vi "Periodic Tasks.vi"(8 "error in":errorcluster) -> ()   [LabVIEW 2013]
doc: "This VI runs in parallel to other tasks. It can contain as many user-defined periodic loops as you need. These can carry out PID or other sorts of timed response."
uses:
  RefnameEnum.ctl
  ActionEnum.ctl
  <vilib>/Rock Robotics/SystemInterfaces/Utilities/FPGA_UtilitiesLED Source.ctl
  <vilib>/Rock Robotics/SystemInterfaces/Utilities/FPGA_UtilitiesLED State.ctl
  TankDriveInstruction.ctl
  Robot Global Data.vi
  <vilib>/Rock Robotics/WPI/Compressor/WPI_CompressorGetSetRefNum.vi
  <vilib>/Rock Robotics/WPI/RobotDrive/WPI_RobotDriveGetSetRefNum.vi
panel:
  out "MainQueue size":i32
  out "TankDriveQueue size":i32
  out "IDNum Diff":i32
  out "MainQueue\nInterval":u32
  out "TankDrive\nInterval":u32
  out "ProcessInput\nInterval":u32
  out "TeleopInterval":i32
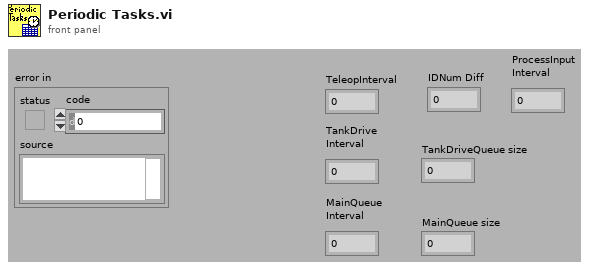
[diagram p1: front panel]
types:
  T1 = typedef "ActionEnum.ctl" = enum16{"Init", "SetValue"}
  T2 = typedef "RefnameEnum.ctl" = enum16{"FireLauncher", "Climber", "Shield", "TankDrive", "DriveEncoderL", "DriveEncoderR", "LauncherMotorRPM", "LauncherEncoderAnalog", "LauncherEncoderRPM", "ShooterLS", "DriveAlignLSLeft", "DriveAlignLSRight", "ClimbingLS", "LauncherEncoderAngle", "LauncherMotorAngle", "Gamepad1", "Gamepad2", "Compressor", "ClimbWeightSol3", "ClimbWeightSol4"}
  T3 = typedef "WPI_SolenoidDevRef.ctl" = cluster{"DevStatus":errorcluster, "Solenoid Module":T4, "Forward Solenoid Channel":T5, "Reverse Solenoid Channel":T5}
  T4 = typedef "FPGA_TypedefSolenoidModule.ctl" = enum16{"Solenoid Module 1", "Solenoid Module 2"}
  T5 = typedef "WPI_SolenoidChannel.ctl" = enum8{"Solenoid 1", "Solenoid 2", "Solenoid 3", "Solenoid 4", "Solenoid 5", "Solenoid 6", "Solenoid 7", "Solenoid 8", "Invalid"}
  T6 = typedef "WPI_RobotDriveDevRef.ctl" = cluster{"DevStatus":errorcluster, "Motors[]":T7[], "Square Inputs":bool, "Max Output":dbl, "Isochronous":bool}
  T7 = typedef "WPI_MotorControlDeviceRef.ctl" = cluster{"DeviceStatus":errorcluster, "Type":enum16{"PWM", "CAN"}, "PWM":cluster{"Digital Module":T8, "PWM Channel":T9, "DeadBand":T10}, "CAN":cluster{"Device Number":u8, "Control Mode":T11, "Semaphore":T12, "Max Vout":dbl}, "Invert":bool, "TransformRef":T13, "InvTransformRef":T13}
  T8 = typedef "FPGA_TypedefDigitalModule.ctl" = enum16{"Digital Module 1", "Digital Module 2"}
  T9 = typedef "FPGA_DIOPWMChannel.ctl" = enum8{"PWM 1", "PWM 2", "PWM 3", "PWM 4", "PWM 5", "PWM 6", "PWM 7", "PWM 8", "PWM 9", "PWM 10", "Invalid"}
  T10 = typedef "WPI_PWMDeadband.ctl" = cluster{"Name":string, "maxPositivePwm":i32, "minPositivePwm":i32, "centerPwm":i32, "maxNegativePwm":i32, "minNegativePwm":i32, "angularRange":u16}
  T11 = typedef "WPI_CANJaguar_ControlMode.ctl" = enum8{"Percent VBus", "Current", "Speed", "Position", "Voltage"}
  T12 = typedef "Semaphore RefNum" = refnum<k1>
  T13 = typedef "WPI_PWMTransform_ConPane.ctl" = refnum<vi>
  T14 = typedef "WPI_CompressorDevRef.ctl" = cluster{"DevStatus":errorcluster, "DigitalInputDevRef":T15, "RelayDevRef":T17}
  T15 = typedef "WPI_DigitalInputDevRef.ctl" = cluster{"DevStatus":errorcluster, "DIO Channel":T16, "Digital Module":T8}
  T16 = typedef "FPGA_DIOChannel.ctl" = enum8{"DIO 1", "DIO 2", "DIO 3", "DIO 4", "DIO 5", "DIO 6", "DIO 7", "DIO 8", "DIO 9", "DIO 10", "DIO 11", "DIO 12", "DIO 13", "DIO 14", "Invalid"}
  T17 = typedef "WPI_RelayDevRef.ctl" = cluster{"DevStatus":errorcluster, "Relay Channel":T18, "Digital Module":T8, "Relay Direction":T19}
  T18 = typedef "FPGA_DIORelayChannel.ctl" = enum8{"Relay 1", "Relay 2", "Relay 3", "Relay 4", "Relay 5", "Relay 6", "Relay 7", "Relay 8", "Invalid"}
  T19 = typedef "WPI_RelayDirection.ctl" = enum16{"Both directions", "Forward only", "Reverse only"}
  T20 = typedef "QueueInstruction.ctl" = cluster{"Data":variant, "Subsystem":T21, "Action":T1}
  T21 = typedef "SubsystemEnum.ctl" = enum16{"TankDrive", "FirePneumatic", "Climber", "ClimbWeight", "ShooterAngle"}
  T22 = typedef "TankDriveInstruction.ctl" = cluster{"LeftMotorValue":dbl, "RightMotorValue":dbl, "HalfSpeed":bool}
  T23 = typedef "FPGA_UtilitiesLED State.ctl" = enum16{"Off", "On", "Toggle"}
  T24 = typedef "FPGA_UtilitiesLED Source.ctl" = enum16{"User LED", "FPGA LED"}
  T25 = typedef "TeleopData.ctl" = cluster{"cTankDriveLeft":dbl, "cTankDriveRight":dbl, "cHalfSpeed":bool, "cClimbWeight":bool, "cClimbStart":bool, "cRpmControl":dbl, "cAngleControl":dbl, "cQuickShoot":bool, "cLauncherWheel":bool, "cFirePneumatic":bool, "cPresetLow":bool, "cPresetHigh":bool, "cPresetClimbLow":bool, "cPresetClimbHigh":bool, "cLauncherAngle":bool, "cResetAngleEncoder":bool, "IDNum":i32, "TeleopInterval":i32}
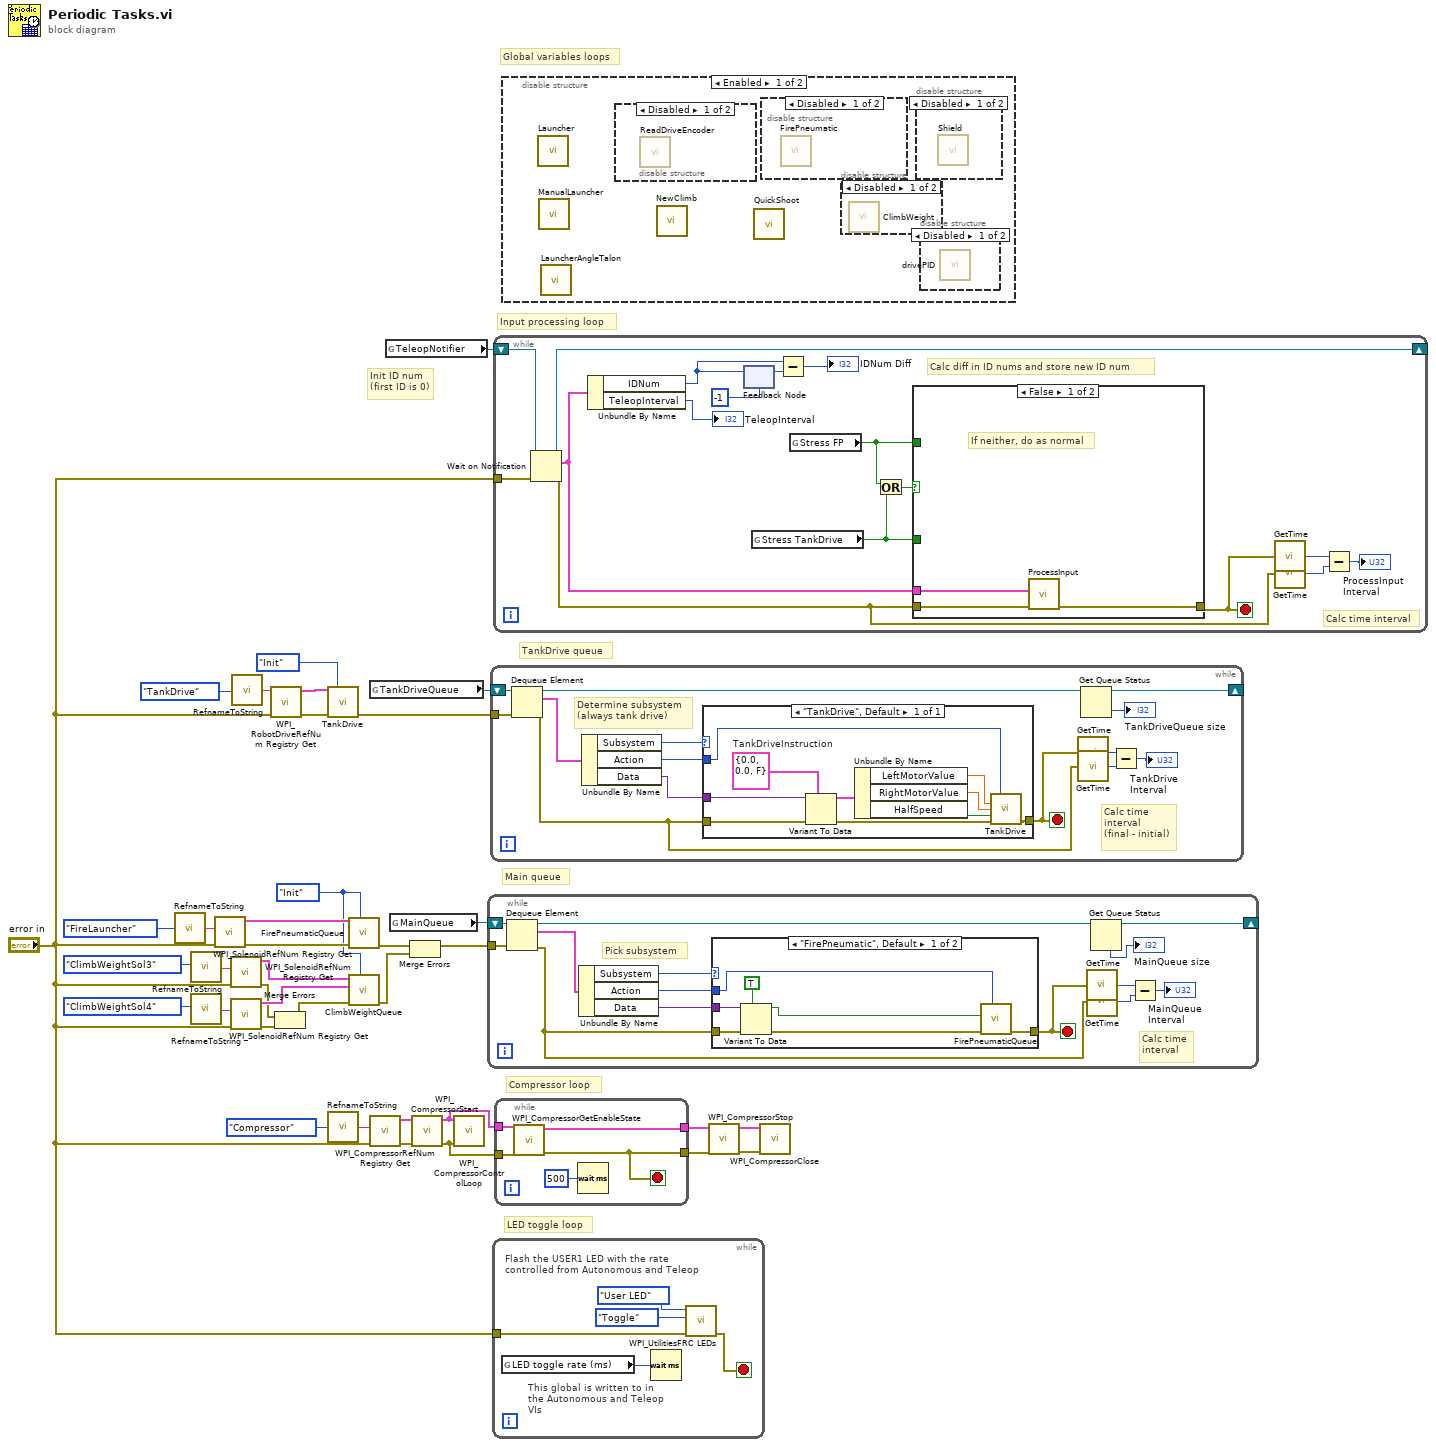
[diagram p0: block diagram]
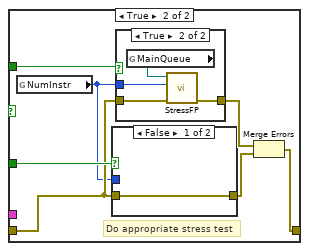
[diagram p2: hidden frame]
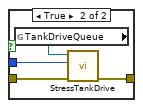
[diagram p3: hidden frame]
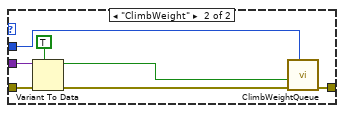
[diagram p5: hidden frame]
diagram:
  w2 = ActionEnum."Init" ("Action")
  # "Init ID num\n(first ID is 0)"
  # "Global variables loops"
  # "LED toggle loop"
  # "Compressor loop"
  # "Main queue"
  # "Input processing loop"
  # "TankDrive queue"
  n1 = call "RefnameToString.vi"("Enum"=RefnameEnum."FireLauncher") -> ("Refname"=w25:string)
  n2 = call "RefnameToString.vi"("Enum"=RefnameEnum."ClimbWeightSol3") -> ("Refname"=w11:string)
  n3 = call "RefnameToString.vi"("Enum"=RefnameEnum."ClimbWeightSol4") -> ("Refname"=w9:string)
  n4 = call <vilib>:"WPI_SolenoidRefNum Registry Get.vi"("error in (no error)"="error in", "refnum name"=w25) -> ("error out"=w18:errorcluster, "SolenoidDevRef"=w19:T3)  [unwired: 8 in]
  n5 = call <vilib>:"WPI_SolenoidRefNum Registry Get.vi"("error in (no error)"="error in", "refnum name"=w11) -> ("error out"=w4:errorcluster, "SolenoidDevRef"=w7:T3)  [unwired: 8 in]
  n6 = call <vilib>:"WPI_SolenoidRefNum Registry Get.vi"("error in (no error)"="error in", "refnum name"=w9) -> ("error out"=w5:errorcluster, "SolenoidDevRef"=w6:T3)  [unwired: 8 in]
  n7 = call "RefnameToString.vi"("Enum"=RefnameEnum."TankDrive") -> ("Refname"=w30:string)
  n8 = call <vilib>:"WPI_RobotDriveRefNum Registry Get.vi"("error in (no error)"="error in", "refnum name"=w30) -> ("error out"=w21:errorcluster, "RobotDriveDevRef"=w22:T6)  [unwired: 8 in]
  n9 = Merge Errors(w4, w5) -> (w3:errorcluster)
  n10 = call "TankDrive.vi"("RobotDriveDevRef"=w22, "Action"=ActionEnum."Init", "Error In (no error)"=w21) -> ("Error Out"=w20:errorcluster)  [unwired: 12 in]
  n11 = call "RefnameToString.vi"("Enum"=RefnameEnum."Compressor") -> ("Refname"=w32:string)
  n12 = call "FirePneumaticQueue.vi"("Action"=w2, "error in (no error)"=w18, "SolenoidDevRef"=w19) -> ("error out"=w15:errorcluster)  [unwired: 8 in]
  n13 = call "ClimbWeightQueue.vi"("Action"=w2, "error in (no error)"=w3, "ClimbWeightSol4"=w6, "ClimbWeightSol3"=w7) -> ("error out"=w13:errorcluster)  [unwired: 7 in]
  n14 = global read "Robot Global Data.vi" "TankDriveQueue"() -> (w28:refnum<queue>)
  n15 = call <vilib>:"WPI_CompressorRefNum Registry Get.vi"("error in (no error)"="error in", "refnum name"=w32) -> ("error out"=w24:errorcluster, "CompressorDevRef"=w37:T14)  [unwired: 8 in]
  n16 = global read "Robot Global Data.vi" "TeleopNotifier"() -> (w29:refnum<notifier>)
  n17 = global read "Robot Global Data.vi" "MainQueue"() -> (w27:refnum<queue>)
  n18 = Merge Errors(w15, w13) -> (w14:errorcluster)
  n19 = call <vilib>:"WPI_CompressorStart.vi"("error in (no error)"=w24, "CompressorDevRef"=w37) -> ("error out"=w23:errorcluster, "CompressorDevRef"=w36:T14)  [unwired: 8 in]
  n20 = call <vilib>:"WPI_CompressorControlLoop.vi"("error in (no error)"=w23, "CompressorDevRef"=w36) -> ()  [unwired: 10 in]
  n21 = while {
    shift-right: [w41] -> _
    shift-left: w27 -> [w51]
    tunnel: w14 -> [w49]
    stop <- w44 stop-if-true
    # "Calc time\ninterval"
    # "Pick subsystem"
    n22 = Dequeue Element(queue=w51, error in (no error)=w49) -> (queue out=w42:refnum<queue>, element=w50:T20, error out=w43:errorcluster)  [unwired: 1 in, 1 out]
    n23 = Unbundle By Name(w50) -> ("Subsystem"=w48:T21, "Action"=w38:T1, "Data"=w39:variant)
    n24 = case shown="\"FirePneumatic\", Default" w48 {
      tunnel: w43 -> [w54 w64]
      tunnel: [w57 w65] -> w44
      tunnel: w39 -> [w55 w62]
      tunnel: w38 -> [w52 w59]
      frame "FirePneumatic", Default {
        n25 = Variant To Data(error in=w54, type=TRUE, Variant=w55) -> (data=w56:bool, error out=w53:errorcluster)
        n26 = call "FirePneumaticQueue.vi"("Action"=w52, "error in (no error)"=w53, "On/off?"=w56) -> ("error out"=w57:errorcluster)  [unwired: 8 in]
      }
      frame "ClimbWeight" {
        n27 = Variant To Data(error in=w64, type=TRUE, Variant=w62) -> (data=w60:bool, error out=w63:errorcluster)
        n28 = call "ClimbWeightQueue.vi"("Action"=w59, "error in (no error)"=w63, "Swing Out?"=w60) -> ("error out"=w65:errorcluster)  [unwired: 8 in]
      }
    }
    n29 = call "GetTime.vi"("error in"=w44) -> ("Time"=w46:u32)
    n30 = call "GetTime.vi"("error in"=w43) -> ("Time"=w47:u32)
    n31 = Get Queue Status(queue=w42) -> (queue out=w41:refnum<queue>, # elements in queue=→"MainQueue size":i32)  [unwired: 2 in, 6 out]
    n32 = Subtract(x=w46, y=w47) -> (x-y=→"MainQueue\nInterval":u32)
  }
  n33 = while {
    shift-right: [w69] -> _
    shift-left: w28 -> [w79]
    tunnel: w20 -> [w76]
    stop <- w74 stop-if-true
    # "Calc time\ninterval\n(final - initial)"
    # "Determine subsystem\n(always tank drive)"
    n34 = Dequeue Element(queue=w79, error in (no error)=w76) -> (queue out=w70:refnum<queue>, element=w78:T20, error out=w75:errorcluster)  [unwired: 1 in, 1 out]
    n35 = Unbundle By Name(w78) -> ("Subsystem"=w77:T21, "Action"=w66:T1, "Data"=w67:variant)
    n36 = case shown="\"TankDrive\", Default" w77 {
      tunnel: w75 -> [w86]
      tunnel: [w85] -> w74
      tunnel: w67 -> [w81]
      tunnel: w66 -> [w80]
      frame "TankDrive", Default {
        w89 = T22 {"LeftMotorValue"=0.0, "RightMotorValue"=0.0, "HalfSpeed"=FALSE}  # TankDriveInstruction
        n37 = Variant To Data(error in=w86, type=w89, Variant=w81) -> (data=w88:T22, error out=w87:errorcluster)
        n38 = Unbundle By Name(w88) -> ("LeftMotorValue"=w82:dbl, "RightMotorValue"=w83:dbl, "HalfSpeed"=w84:bool)
        n39 = call "TankDrive.vi"("Action"=w80, "Left Motor Value"=w82, "Right Motor Value"=w83, "HalfSpeed"=w84, "Error In (no error)"=w87) -> ("Error Out"=w85:errorcluster)  [unwired: 10 in]
      }
    }
    n40 = call "GetTime.vi"("error in"=w74) -> ("Time"=w72:u32)
    n41 = call "GetTime.vi"("error in"=w75) -> ("Time"=w71:u32)
    n42 = Get Queue Status(queue=w70) -> (queue out=w69:refnum<queue>, # elements in queue=→"TankDriveQueue size":i32)  [unwired: 2 in, 6 out]
    n43 = Subtract(x=w72, y=w71) -> (x-y=→"TankDrive\nInterval":u32)
  }
  n44 = while {
    tunnel: "error in" -> [w91]
    stop <- w90 stop-if-true
    # "This global is written to in the Autonomous and Teleop VIs"
    # "Flash the USER1 LED with the rate controlled from Autonomous and Teleop"
    n45 = global read "Robot Global Data.vi" "LED toggle rate (ms)"() -> (w92:u32)
    n46 = Wait (ms)(milliseconds to wait=w92) -> ()  [unwired: 1 out]
    n47 = call <vilib>:"WPI_UtilitiesFRC LEDs.vi"("error in (no error)"=w91, "State"=FPGA_UtilitiesLED_State."Toggle", "LED Type"=FPGA_UtilitiesLED_Source."User LED") -> ("error out"=w90:errorcluster)  [unwired: 8 out]
  }
  n48 = while {
    shift-right: [w110] -> _
    shift-left: w29 -> [w111]
    tunnel: "error in" -> [w109]
    stop <- w100 stop-if-true
    # "Calc diff in ID nums and store new ID num"
    # "Calc time interval"
    n49 = Wait on Notification(notifier=w111, error in (no error)=w109) -> (notifier out=w110:refnum<notifier>, notification=w108:T25, error out=w99:errorcluster)  [unwired: 2 in, 1 out]
    n50 = Unbundle By Name(w108) -> ("IDNum"=w97:i32, "TeleopInterval"=→"TeleopInterval":i32)
    n51 = feedback-in #1(w97) -> ()
    n52 = feedback #1(-1) -> (w96:i32)
    n53 = global read "Robot Global Data.vi" "Stress TankDrive"() -> (w102:bool)
    n54 = Subtract(x=w97, y=w96) -> (x-y=→"IDNum Diff":i32)
    n55 = global read "Robot Global Data.vi" "Stress FP"() -> (w101:bool)
    n56 = Or(x=w101, y=w102) -> (x .or. y?=w103:bool)
    n57 = case shown="False" w103 {
      tunnel: w108 -> [w114 _]
      tunnel: [w113 w115] -> w100
      tunnel: w99 -> [w112 w119]
      tunnel: w102 -> [_ w120]
      tunnel: w101 -> [_ w121]
      frame False {
        # "If neither, do as normal"
        n58 = call "ProcessInput.vi"("Error In (no error)"=w112, "TeleopData"=w114) -> ("Error Out"=w113:errorcluster)  [unwired: 9 in]
      }
      frame True {
        # "Do appropriate stress test"
        n59 = global read "Robot Global Data.vi" "NumInstr"() -> (w118:i32)
        n60 = case shown="False" w120 {
          tunnel: [w122 w125] -> w117
          tunnel: w119 -> [w122 w124]
          tunnel: w118 -> [_ w123]
          frame False {
          }
          frame True {
            n61 = global read "Robot Global Data.vi" "TankDriveQueue"() -> (w126:refnum<queue>)
            n62 = call "StressTankDrive.vi"("error in (no error)"=w124, "Num instructions"=w123, "TankDriveQueue"=w126) -> ("error out"=w125:errorcluster)  [unwired: 8 in]
          }
        }
        n63 = case shown="True" w121 {
          tunnel: [w127 w130] -> w116
          tunnel: w119 -> [w127 w129]
          tunnel: w118 -> [_ w128]
          frame False {
          }
          frame True {
            n64 = global read "Robot Global Data.vi" "MainQueue"() -> (w131:refnum<queue>)
            n65 = call "StressFP.vi"("error in (no error)"=w129, "Num instructions"=w128, "MainQueue"=w131) -> ("error out"=w130:errorcluster)  [unwired: 8 in]
          }
        }
        n66 = Merge Errors(w116, w117) -> (w115:errorcluster)
      }
    }
    n67 = call "GetTime.vi"("error in"=w100) -> ("Time"=w106:u32)
    n68 = call "GetTime.vi"("error in"=w99) -> ("Time"=w98:u32)
    n69 = Subtract(x=w106, y=w98) -> (x-y=→"ProcessInput\nInterval":u32)
  }
  n70 = while {
    tunnel: w36 -> [w136]
    tunnel: [w134] -> w35
    tunnel: w23 -> [w133]
    tunnel: [w132] -> w17
    stop <- w132 stop-if-true
    n71 = call <vilib>:"WPI_CompressorGetEnableState.vi"("error in (no error)"=w133, "CompressorDevRef"=w136) -> ("error out"=w132:errorcluster, "CompressorDevRef"=w134:T14)  [unwired: 8 out]
    n72 = Wait (ms)(milliseconds to wait=u32 500) -> ()  [unwired: 1 out]
  }
  n73 = disable-structure shown="Enabled" {
    frame Enabled {
      n74 = call "Launcher.vi"() -> ()  [unwired: 12 in]
      n75 = call "ManualLauncher.vi"() -> ()  [unwired: 12 in]
      n76 = call "LauncherAngleTalon.vi"() -> ()  [unwired: 12 in]
      n77 = disable-structure shown="Disabled" {
        frame Disabled {
          n78 = call "ReadDriveEncoder.vi"() -> ()  [unwired: 12 in]
        }
        frame Enabled {
        }
      }
      n79 = call "NewClimb.vi"() -> ()  [unwired: 12 in]
      n80 = call "QuickShoot.vi"() -> ()  [unwired: 12 in]
      n81 = disable-structure shown="Disabled" {
        frame Disabled {
          n82 = call "FirePneumatic.vi"() -> ()  [unwired: 12 in]
        }
        frame Enabled {
        }
      }
      n83 = disable-structure shown="Disabled" {
        frame Disabled {
          n84 = call "ClimbWeight.vi"() -> ()  [unwired: 12 in]
        }
        frame Enabled {
        }
      }
      n85 = disable-structure shown="Disabled" {
        frame Disabled {
          n86 = call "Shield.vi"() -> ()  [unwired: 12 in]
        }
        frame Enabled {
        }
      }
      n87 = disable-structure shown="Disabled" {
        frame Disabled {
          n88 = call "drivePID.vi"() -> ()  [unwired: 12 in]
        }
        frame Enabled {
        }
      }
    }
    frame Disabled {
    }
  }
  n89 = call <vilib>:"WPI_CompressorStop.vi"("error in (no error)"=w17, "CompressorDevRef"=w35) -> ("error out"=w16:errorcluster, "CompressorDevRef"=w34:T14)  [unwired: 8 out]
  n90 = call <vilib>:"WPI_CompressorClose.vi"("error in (no error)"=w16, "CompressorDevRef"=w34) -> ()  [unwired: 10 out]
